vi "Frequency to phase word DBL.vi"(6 "Synchonous":bool, 9 "DDS modulus":i64=4294967296 format="0x%x (%d)", 10 "DDS clock":dbl=125000000.0 format="%_13p", 11 "Frequency":dbl format="%#_15p") -> (2 "Actual frequency":dbl format="%#_12pHz", 3 "Phase word":u64=1717987 format="0x%x (%d) 0b%b")   [LabVIEW 2019]
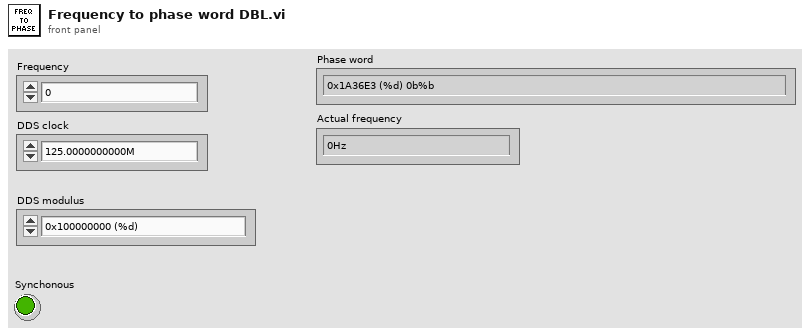
[diagram p1: front panel]
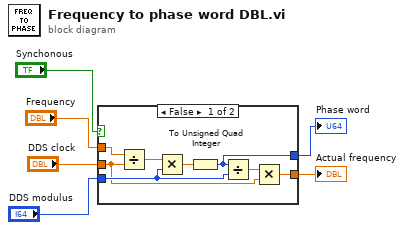
[diagram p0: block diagram]
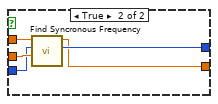
[diagram p2: hidden frame]
diagram:
  n1 = case shown="False" "Synchonous" {
    tunnel: "Frequency" -> [w12 w16]
    tunnel: [w11 w19] -> w5
    tunnel: "DDS modulus" -> [w10 w15]
    tunnel: "DDS clock" -> [w8 w17]
    tunnel: [w7 w18] -> w2
    frame False {
      n2 = Divide(x=w12, y=w8) -> (x/y=w14:dbl)
      n3 = Multiply(x=w14, y=w10) -> (x*y=w13:dbl)
      n4 = To Unsigned Quad Integer(1:w13) -> (0:w11:u64)
      n5 = Divide(x=w11, y=w10) -> (x/y=w9:dbl)
      n6 = Multiply(x=w9, y=w8) -> (x*y=w7:dbl)
    }
    frame True {
      n7 = call "Find Syncronous Frequency.vi"("DDS clock"=w17, "DDS modulus"=w15, "Frequency"=w16) -> ("Frequency word"=w19:i64, "Actual frequency"=w18:dbl)  [unwired: 5 in, 2 out]
    }
  }
  "Phase word" <- w5
  "Actual frequency" <- w2
